vi "RT Check to Activate.vi"(11 "All Notifier":T1) -> ()   [LabVIEW 2022 SP3]
uses:
  RT Controls/RT All Notifer.ctl
  RT Sequence Control.ctl
  RT Controls/RT All Loop Status.ctl
  RT Sub VI's/RT Global.vi
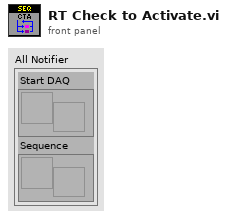
[diagram p1: front panel]
types:
  T1 = typedef "RT All Notifer.ctl" = cluster{"Start DAQ":refnum<notifier>, "Sequence":refnum<notifier>}
  T2 = cluster{"Sequence":refnum<notifier>, "Seq data":cluster{"AO":cluster{"CDT":dbl, "Range":dbl, "Component ID":string}[], "DO":cluster{"CDT":dbl, "Position":bool, "Component ID":string}[], "Launch Time":timestamp}}
  T3 = typedef "RT Sequence Control.ctl" = enum16{"Initialize", "Polevent", "Ready for Seq", "Hold", "Abort Seq", "Exit"}
  T4 = typedef "RT All Loop Status.ctl" = enum16{"AI", "AO", "DI", "DO", "TC", "Strain", "ACC", "RT", "Log", "Seq", "Sync"}
  T5 = enum16{"Init", "Read 'All'", "Read 'n'", "Read '1'", "Write '1'", "Write 'n'", "Write 'All'"}
  T6 = cluster{"AO":cluster{"CDT":dbl, "Range":dbl, "Component ID":string}[], "DO":cluster{"CDT":dbl, "Position":bool, "Component ID":string}[], "Launch Time":timestamp}
  T7 = cluster{"CDT":dbl, "Position":bool, "Component ID":string}[]
  T8 = cluster{"CDT":dbl, "Range":dbl, "Component ID":string}[]
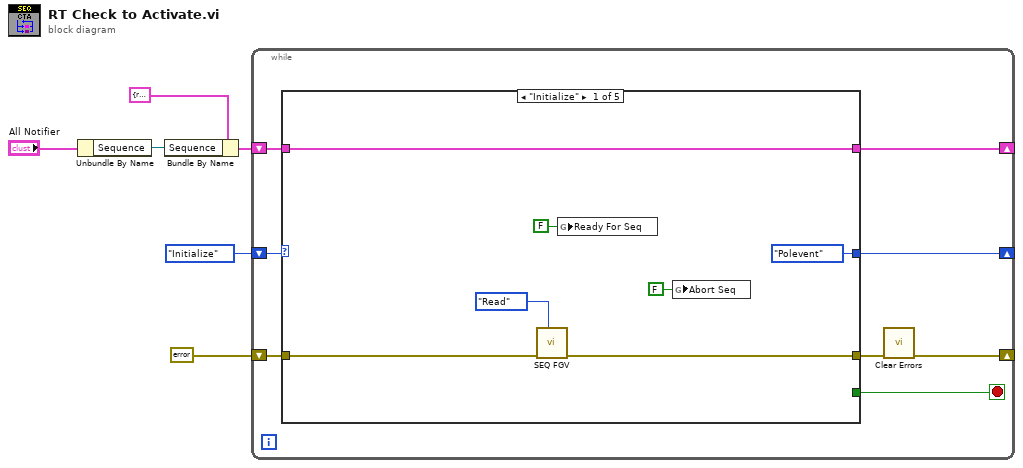
[diagram p0: block diagram]
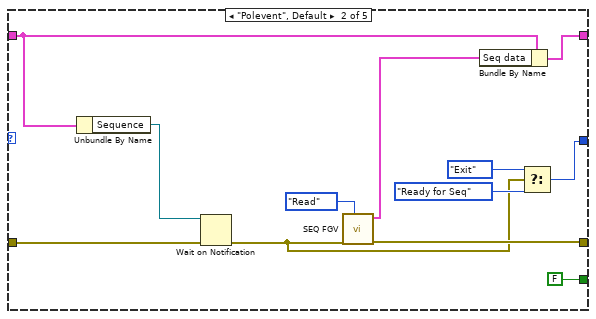
[diagram p2: hidden frame]
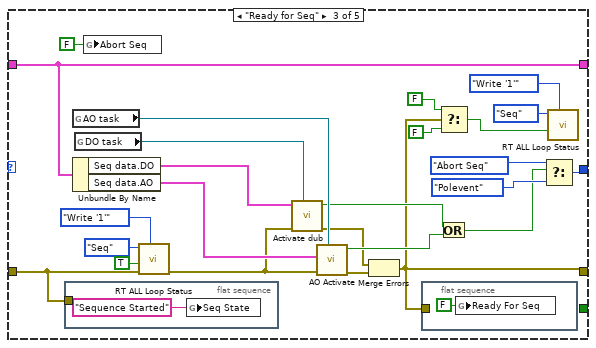
[diagram p3: hidden frame]
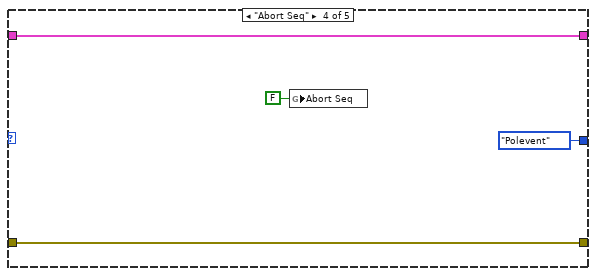
[diagram p4: hidden frame]
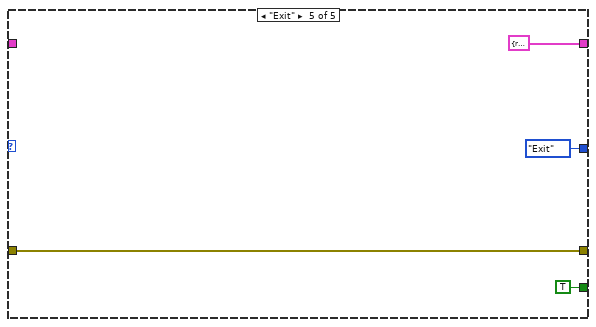
[diagram p5: hidden frame]
diagram:
  n1 = Unbundle By Name("All Notifier") -> ("Sequence"=w2:refnum<notifier>)
  n2 = Bundle By Name(cluster=T2 {"Sequence"=refnum, "Seq data"={"AO"=[], "DO"=[], "Launch Time"=timestamp(0 s since 1904-01-01)}}, "Sequence"=w2) -> (w4:T2)
  n3 = while {
    shift-right: [w12] -> _
    shift-left: RT_Sequence_Control."Initialize" ("Enum") -> [w13]
    shift-right: [w9] -> _
    shift-left: errorcluster {"status"=FALSE, "code"=0, "source"=""} ("error in (no error)") -> [w11]
    shift-right: [w8] -> _
    shift-left: w4 -> [w7]
    stop <- w14 stop-if-true
    n4 = case shown="\"Initialize\"" w13 {
      tunnel: [_ FALSE _ _ TRUE] -> w14
      tunnel: [RT_Sequence_Control."Polevent" ("Enum") w24 w56 RT_Sequence_Control."Polevent" ("Enum") RT_Sequence_Control."Exit" ("Enum")] -> w12
      tunnel: w11 -> [w21 w32 w45 w62 w66]
      tunnel: [w20 w23 w35 w62 w66] -> w10
      tunnel: [w18 w29 w58 w64 T2 {"Sequence"=refnum, "Seq data"={"AO"=[], "DO"=[], "Launch Time"=timestamp(0 s since 1904-01-01)}}] -> w8
      tunnel: w7 -> [w18 w28 w58 w64 _]
      frame "Initialize" {
        n5 = call "SEQ FGV.vi"("Enum"=enum16{"Read", "Write"}."Read", "error in (no error)"=w21) -> ("error out"=w20:errorcluster)  [unwired: 8 in, 1 out]
        n6 = global write "RT Global.vi" "Ready For Seq"(FALSE ("Ready For Seq")) -> ()
        n7 = global write "RT Global.vi" "Abort Seq"(FALSE ("Abort Seq")) -> ()
      }
      frame "Polevent", Default {
        n8 = Unbundle By Name(w28) -> ("Sequence"=w31:refnum<notifier>)
        n9 = Wait on Notification(notifier=w31, error in (no error)=w32) -> (error out=w22:errorcluster)  [unwired: 2 in, 3 out]
        n10 = call "SEQ FGV.vi"("Enum"=enum16{"Read", "Write"}."Read", "error in (no error)"=w22) -> ("error out"=w23:errorcluster, "Seq data out"=w27:T6)  [unwired: 8 in]
        n11 = Bundle By Name(cluster=w28, "Seq data"=w27) -> (w29:T2)
        n12 = Select(t=RT_Sequence_Control."Exit" ("Enum"), s=w22, f=RT_Sequence_Control."Ready for Seq" ("Enum")) -> (s? t:f=w24:T3)
      }
      frame "Ready for Seq" {
        n13 = flat-sequence {
          tunnel: w45 -> [_]
          frame #0 {
            n14 = global write "RT Global.vi" "Seq State"("Sequence Started" ("Seq State")) -> ()
          }
        }
        n15 = global read "RT Global.vi" "AO task"() -> (w42:refnum<k21>)
        n16 = Unbundle By Name(w58) -> ("Seq data.DO"=w41:T7, "Seq data.AO"=w57:T8)
        n17 = global read "RT Global.vi" "DO task"() -> (w40:refnum<k21>)
        n18 = global write "RT Global.vi" "Abort Seq"(FALSE ("Abort Seq")) -> ()
        n19 = call "RT ALL Loop Status.vi"("Option"=T5."Write '1'", "error in (no error)"=w45, "Status"=TRUE, "Loop"=RT_All_Loop_Status."Seq") -> ("error out"=w39:errorcluster)  [unwired: 5 in, 2 out]
        n20 = call "Activate dub.vi"("DO Task"=w40, "error constant"=w39, "DO"=w41) -> ("error out"=w34:errorcluster, "Abort"=w38:bool)  [unwired: 7 in]
        n21 = call "AO Activate.vi"("AO Task"=w42, "error constant"=w39, "AO"=w57) -> ("error out"=w44:errorcluster, "Abort"=w37:bool)  [unwired: 7 in]
        n22 = Merge Errors(w34, w44) -> (w35:errorcluster)
        n23 = flat-sequence {
          tunnel: w35 -> [_]
          frame #0 {
            n24 = global write "RT Global.vi" "Ready For Seq"(FALSE ("Ready For Seq")) -> ()
          }
        }
        n25 = Select(t=FALSE ("Status"), s=w35, f=FALSE) -> (s? t:f=w47:bool)
        n26 = Or(x=w38, y=w37) -> (x .or. y?=w36:bool)
        n27 = Select(t=RT_Sequence_Control."Abort Seq" ("Enum"), s=w36, f=RT_Sequence_Control."Polevent" ("Enum")) -> (s? t:f=w56:T3)
        n28 = call "RT ALL Loop Status.vi"("Option"=T5."Write '1'", "Status"=w47, "Loop"=RT_All_Loop_Status."Seq") -> ()  [unwired: 6 in, 3 out]
      }
      frame "Abort Seq" {
        n29 = global write "RT Global.vi" "Abort Seq"(FALSE ("Abort Seq")) -> ()
      }
      frame "Exit" {
      }
    }
    n30 = call <vilib>:"Clear Errors.vi"("error in (no error)"=w10) -> ("error out"=w9:errorcluster)  [unwired: 5 in, 1 out]
  }
